vi "Get Mentions Old.vi"(8 "error in":errorcluster, 9 "Mentions to Read (10)":i32=10 min=0 max=200 step=1, 11 "Twitter Handle In":T2={"OAuth Credentials"={"Consumer Key"="", "Signature Method"=enum."HMAC-SHA1", "Token"="", "Version"="", "Token Secret"="", "Consumer Secret"=""}, "since ID"="", "max ID"="", "Screen Name"=""}) -> (0 "error out":errorcluster, 1 "Actual Num of Mentions Read":i32, 2 "Old Mentions Read":T1[](array[typedef]), 3 "Twitter Handle Out":T2={"OAuth Credentials"={"Consumer Key"="", "Signature Method"=enum."HMAC-SHA1", "Token"="", "Version"="", "Token Secret"="", "Consumer Secret"=""}, "since ID"="", "max ID"="", "Screen Name"=""}, 5 "Time Stamp of Oldest Mention":timestamp)   [LabVIEW 2011, in "i3-twitter.lvlib"]
doc: "Get authenticating user's old mentions."
uses:
  i3-twitter.lvlib
  Controls/Twitter Handle.ctl
  i3-oauth/Controls/OAuth Credentials.ctl
  i3-oauth/Controls/Signature Method.ctl
  Controls/Tweet.ctl
  i3-oauth/Controls/HTTP Method.ctl
  i3-json/JSON Parsing/Get Array Value at Index Files/Get Array Value at Index - Object.vi
  i3-json/JSON Parsing/Get Object Parameter Files/Get Object Parameter - String.vi
  i3-json/JSON Parsing/Get Object Parameter Files/Get Object Parameter - Object.vi
  i3-oauth/i3-oauth.lvlib
  <vilib>/httpClient/LabVIEWHTTPClient.lvlib
  i3-json/i3-json.lvlib
panel:
  out "headers":string
  out "body":string
  out "Full URL":string
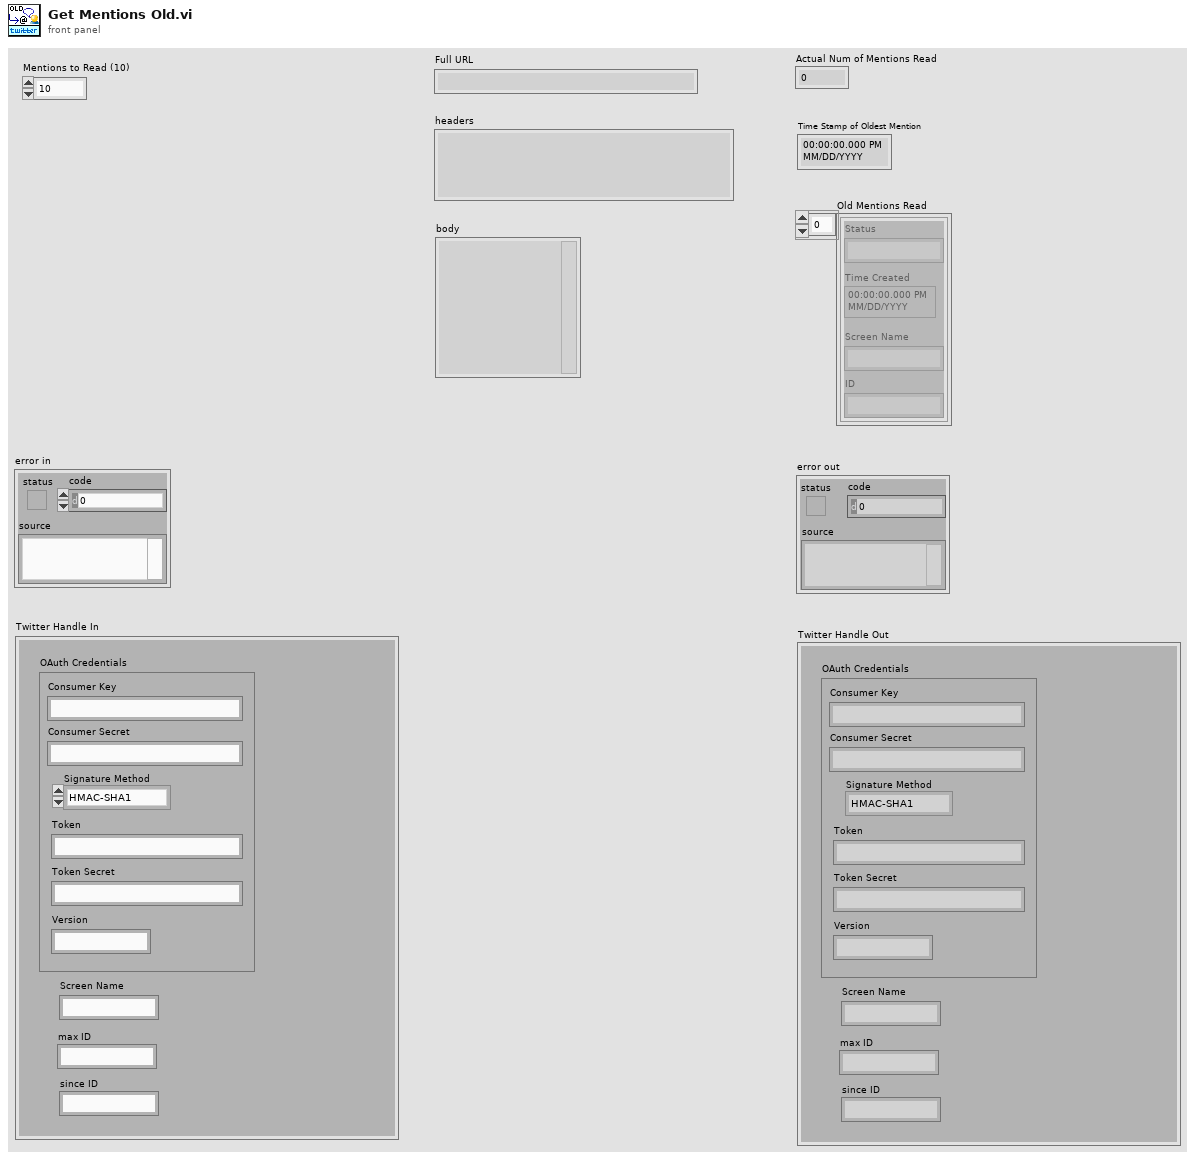
[diagram p1: front panel]
types:
  T1 = typedef "i3-twitter.lvlib/Tweet.ctl" = cluster{"Status":string, "Time Created":timestamp, "Screen Name":string, "ID":string}
  T2 = typedef "i3-twitter.lvlib/Twitter Handle.ctl" = cluster{"OAuth Credentials":T3, "since ID":string, "max ID":string, "Screen Name":string}
  T3 = typedef "i3-oauth.lvlib/OAuth Credentials.ctl" = cluster{"Consumer Key":string, "Signature Method":T4, "Token":string, "Version":string, "Token Secret":string, "Consumer Secret":string}
  T4 = typedef "i3-oauth.lvlib/Signature Method.ctl" = enum16{"HMAC-MD5", "HMAC-SHA1", "HMAC-SHA224", "HMAC-SHA256", "HMAC-SHA384", "HMAC-SHA512"}
  T5 = typedef "i3-oauth.lvlib/HTTP Method.ctl" = enum16{"GET", "POST", "PUT", "DELETE"}
  T6 = typedef "i3-oauth.lvlib/key-value-pairs.ctl" = cluster{"key":string, "value":string}
  T7 = typedef "LabVIEWHTTPClient.lvlib/ClientHandle.ctl" = refnum<k1>
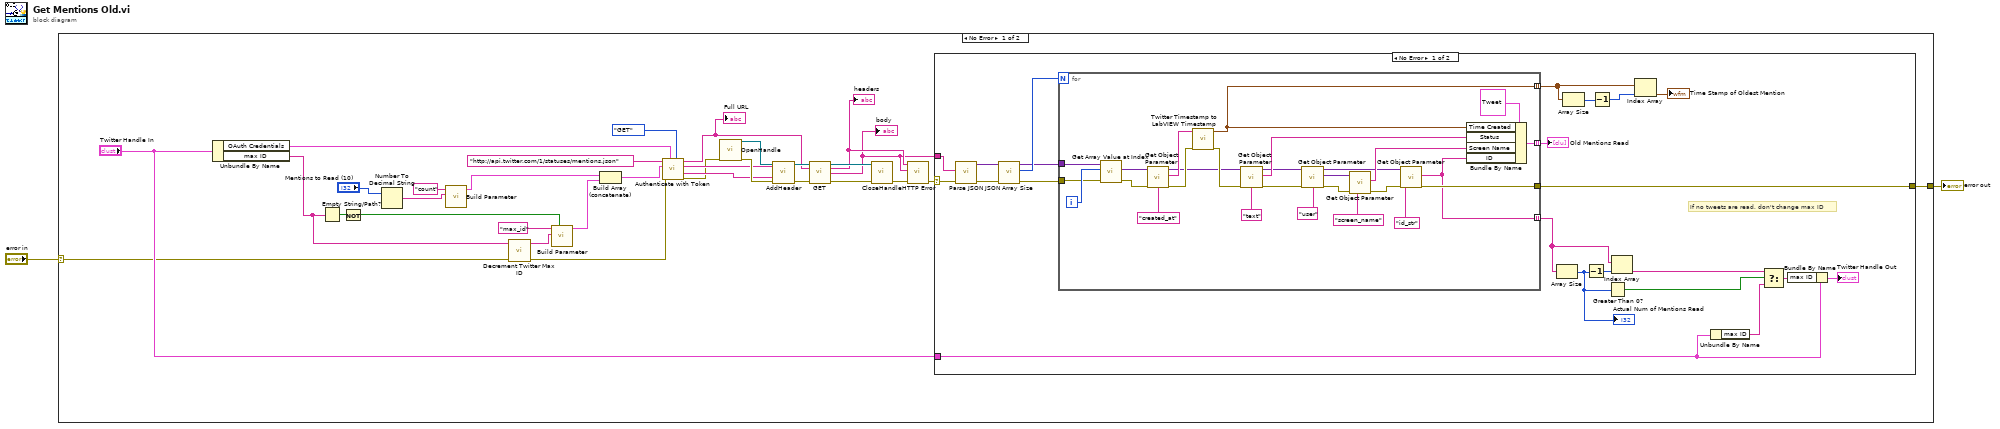
[diagram p0: block diagram]
diagram:
  n1 = case shown="No Error" "error in" {
    selector: "error in" -> [w3 w85]
    tunnel: [w4 w85] -> w2
    frame No Error {
      n2 = Unbundle By Name("Twitter Handle In") -> ("OAuth Credentials"=w8:T3, "max ID"=w6:string)
      n3 = Empty String/Path?(string/path=w6) -> (empty?=w18:bool)
      n4 = Not(x=w18) -> (.not. x?=w14:bool)
      n5 = Number To Decimal String(number="Mentions to Read (10)") -> (decimal integer string=w21:string)  [unwired: 1 in]
      n6 = call "Build Parameter.vi"("Value"=w21, "Key"="count") -> ("Parameter Array"=w7:T6[])  [unwired: 9 in]
      n7 = call "Decrement Twitter Max ID.vi"("error in (no error)"=w3, "ID In"=w6) -> ("error out"=w13:errorcluster, "ID Out"=w15:string)  [unwired: 8 in]
      n8 = call "Build Parameter.vi"("Return Parameter? (T)"=w14, "Value"=w15, "Key"="max_id") -> ("Parameter Array"=w17:T6[])  [unwired: 8 in]
      n9 = Build Array (concatenate)(w7, w17) -> (w20:T6[])
      n10 = call "Authenticate with Token.vi"("HTTP Method"=HTTP_Method."GET", "OAuth Credentials"=w8, "error in (no error)"=w13, "URL Parameters"=w20, "Base URL"="http://api.twitter.com/1/statuses/mentions.json") -> ("error out"=w19:errorcluster, "Header Value"=w26:string, "Header Parameter"=w27:string, "Full URL"=w24:string)  [unwired: 2 in, 1 out]
      "Full URL" <- w24
      n11 = call <vilib>:"OpenHandle.vi"("error in (no error)"=w19) -> ("client handle out"=w33:T7, "error out"=w32:errorcluster)  [unwired: 13 in]
      n12 = call <vilib>:"AddHeader.vi"("client handle"=w33, "header"=w27, "value"=w26, "error in (no error)"=w32) -> ("client handle out"=w31:T7, "error out"=w30:errorcluster)  [unwired: 10 in]
      n13 = call <vilib>:"GET.vi"("client handle"=w31, "url"=w24, "error in (no error)"=w30) -> ("client handle out"=w29:T7, "headers"=w12:string, "body"=w9:string, "error out"=w28:errorcluster)  [unwired: 9 in]
      "body" <- w9
      "headers" <- w12
      n14 = call <vilib>:"CloseHandle.vi"("client handle"=w29, "error in (no error)"=w28) -> ("error out"=w11:errorcluster)  [unwired: 13 in]
      n15 = call "HTTP Error.vi"("error in (no error)"=w11, "Body"=w9, "Header"=w12) -> ("error out"=w10:errorcluster)  [unwired: 6 in, 2 out]
      n16 = case shown="No Error" w10 {
        selector: w10 -> [w44 w84]
        tunnel: "Twitter Handle In" -> [w36 _]
        tunnel: [w41 w84] -> w4
        tunnel: w9 -> [w43 _]
        frame No Error {
          # "If no tweets are read, don't change max ID"
          n17 = call "Parse JSON.vi"("error in (no error)"=w44, "JSON String"=w43) -> ("error out"=w53:errorcluster, "JSON Tree"=w55:variant)  [unwired: 6 in, 2 out]
          n18 = call "JSON Array Size.vi"("error in (no error)"=w53, "JSON Tree In (JSON Array)"=w55) -> ("error out"=w52:errorcluster, "Array Size"=w56:i32, "JSON Tree Passthrough (JSON Array)"=w46:variant)  [unwired: 7 in]
          n19 = for {
            N: w56 -> [_]
            tunnel: [w65] -> w54 mode=indexing
            tunnel: w52 -> [w68]
            tunnel: [w73] -> w51 mode=indexing
            tunnel: [w72] -> w41
            tunnel: w46 -> [w67]
            tunnel: [w66] -> w39 mode=indexing
            i -> [w77]
            n20 = call-poly "Get Array Value at Index.vi"("error in (no error)"=w68, "Index"=w77, "JSON Tree In (JSON Array)"=w67) -> ("error out"=w75:errorcluster, "JSON Object"=w64:variant)  [unwired: 5 in, 2 out]
            n21 = call-poly "Get Object Parameter.vi"("error in (no error)"=w75, "Parameter Name"="created_at", "JSON Tree In (JSON Object)"=w64) -> ("error out"=w62:errorcluster, "String Value"=w61:string, "JSON Tree Out Passthrough"=w60:variant)  [unwired: 5 in, 1 out]
            n22 = call "Twitter Timestamp to LabVIEW Timestamp.vi"("error in"=w62, "Twitter Time Stamp"=w61) -> ("error out"=w71:errorcluster, "LabVIEW Time Stamp"=w66:timestamp)  [unwired: 6 in]
            n23 = call-poly "Get Object Parameter.vi"("error in (no error)"=w71, "Parameter Name"="text", "JSON Tree In (JSON Object)"=w60) -> ("error out"=w59:errorcluster, "String Value"=w69:string, "JSON Tree Out Passthrough"=w58:variant)  [unwired: 5 in, 1 out]
            n24 = call-poly "Get Object Parameter.vi"("error in (no error)"=w59, "Parameter Name"="user", "JSON Tree In (JSON Object)"=w58) -> ("error out"=w74:errorcluster, "JSON Object"=w63:variant, "JSON Tree Out Passthrough"=w57:variant)  [unwired: 5 in, 1 out]
            n25 = call-poly "Get Object Parameter.vi"("error in (no error)"=w74, "Parameter Name"="screen_name", "JSON Tree In (JSON Object)"=w63) -> ("error out"=w70:errorcluster, "String Value"=w80:string)  [unwired: 5 in, 2 out]
            n26 = call-poly "Get Object Parameter.vi"("error in (no error)"=w70, "Parameter Name"="id_str", "JSON Tree In (JSON Object)"=w57) -> ("error out"=w72:errorcluster, "String Value"=w65:string)  [unwired: 5 in, 2 out]
            n27 = Bundle By Name(cluster=T1 {"Status"="", "Time Created"=timestamp(0 s since 1904-01-01), "Screen Name"="", "ID"=""}, "Time Created"=w66, "Status"=w69, "Screen Name"=w80, "ID"=w65) -> (w73:T1)
          }
          "Old Mentions Read" <- w51
          n28 = Array Size(array=w54) -> (size(s)=w49:i32)
          "Actual Num of Mentions Read" <- w49
          n29 = Array Size(array=w39) -> (size(s)=w38:i32)
          n30 = Decrement(x=w49) -> (x-1=w40:i32)
          n31 = Decrement(x=w38) -> (x-1=w37:i32)
          n32 = Greater Than 0?(x=w49) -> (x > 0?=w50:bool)
          n33 = Index Array(array=w54, index=w40) -> (element=w48:string)
          n34 = Index Array(array=w39, index=w37) -> (element=→"Time Stamp of Oldest Mention":timestamp)
          n35 = Unbundle By Name(w36) -> ("max ID"=w35:string)
          n36 = Select(t=w48, s=w50, f=w35) -> (s? t:f=w47:string)
          n37 = Bundle By Name(cluster=w36, "max ID"=w47) -> (→"Twitter Handle Out":T2)
        }
        frame Error {
        }
      }
    }
    frame Error {
    }
  }
  "error out" <- w2
